vi "Main_maszyna.vi"() -> ()   [LabVIEW 2013]
doc: "Use this template to build a standard state machine design pattern. Each state executes code and determines which state to transition to. Contrast this design pattern with the User Interface Event Handler pattern, in which code executes in response to user actions. Contrast this design pattern also with the Queued Message Handler pattern, in which each message handling code can queue zero or more new messages.\nNote: This template does not contain the most recent programming guidelines recommended by National Instruments. For a complete, project-based implementation of the Standard State Machine pattern, use the Create Project dialog box instead of this template."
uses:
  inne pliki/Stany.ctl
  inne pliki/Params.ctl
  inne pliki/Data.ctl
panel:
  out "Warning text":string
  out "Warning":bool
  in  "Temp limits":T1={"Max (25)"=22.0, "Min (0)"=0.0}
  out "Waveform Chart":cluster{"Temperatura":dbl, "Średnia":dbl}(graph)
  in  "Akcje":T2
  out "Stan aktualny":T3
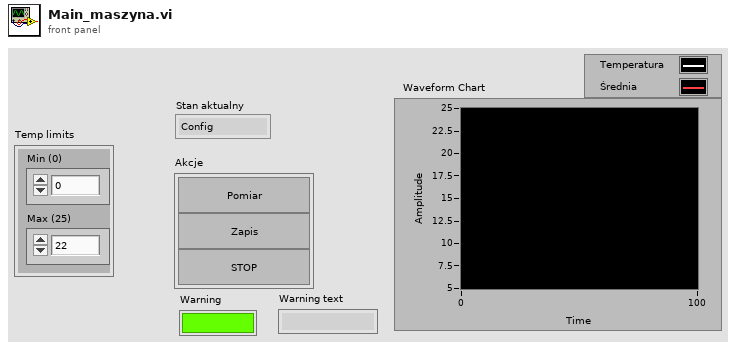
[diagram p1: front panel]
types:
  T1 = typedef "Params.ctl" = cluster{"Max (25)":dbl, "Min (0)":dbl}
  T2 = cluster{"bPomiar":bool, "bZapis":bool, "bSTOP":bool}
  T3 = typedef "Stany.ctl" = enum16{"Config", "IDLE", "Measure", "Analyze", "Display", "STOP", "Save"}
  T4 = typedef "Data.ctl" = cluster{"Temperatura":dbl, "Średnia":dbl, "Warning":bool, "Warning text ":string, "Temp limits":T1}
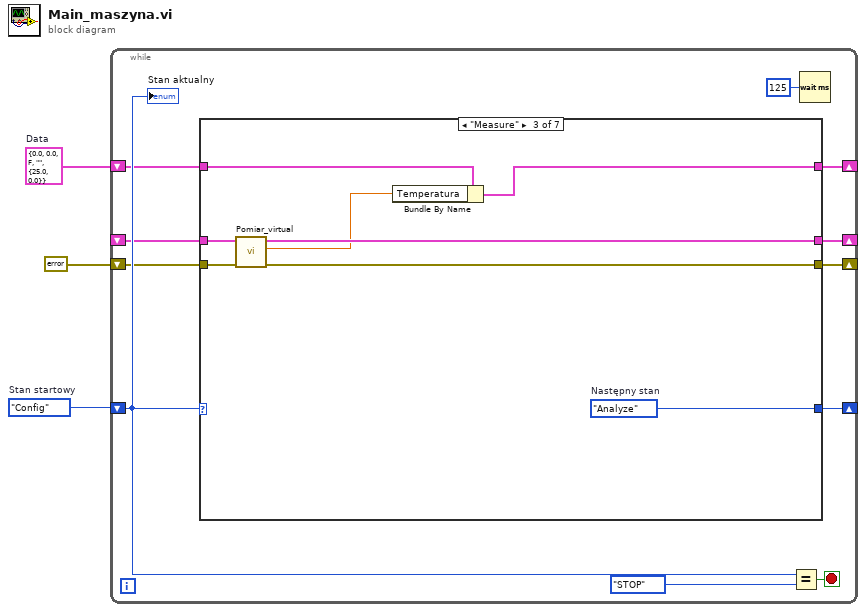
[diagram p0: block diagram]
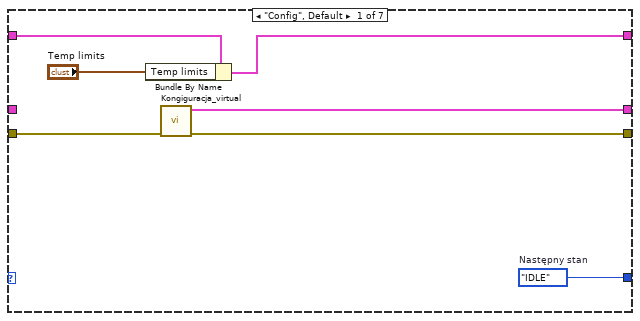
[diagram p2: hidden frame]
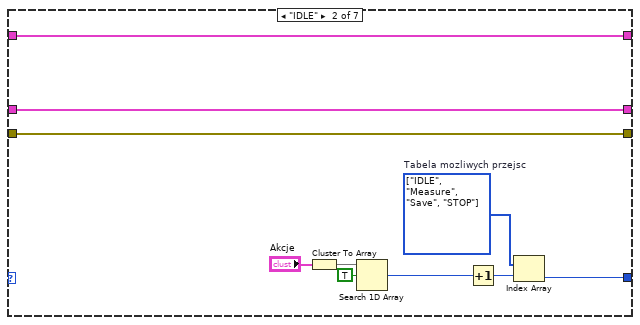
[diagram p3: hidden frame]
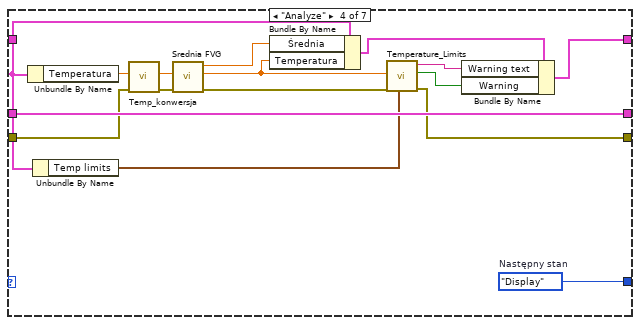
[diagram p4: hidden frame]
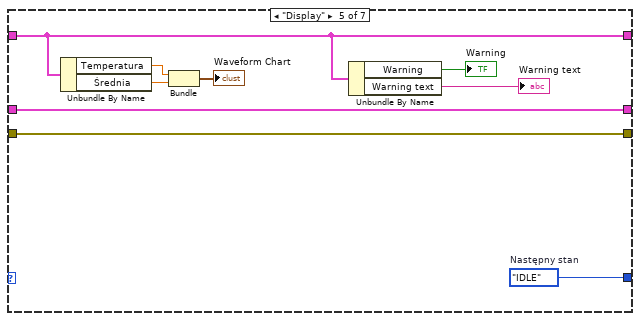
[diagram p5: hidden frame]
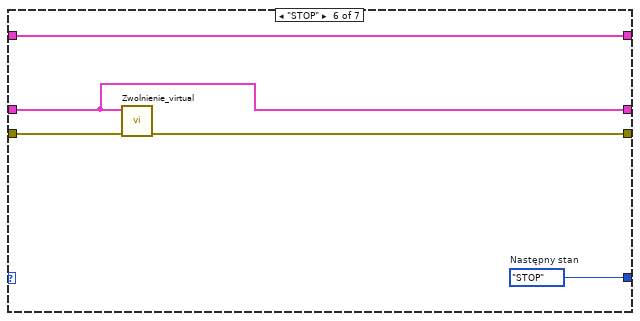
[diagram p6: hidden frame]
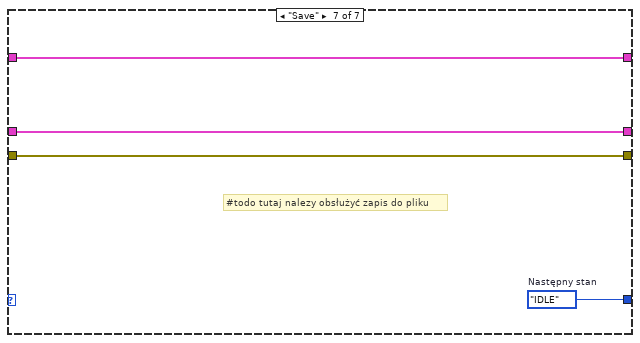
[diagram p7: hidden frame]
diagram:
  w2 = T4 {"Temperatura"=0.0, "Średnia"=0.0, "Warning"=FALSE, "Warning text "="", "Temp limits"={"Max (25)"=25.0, "Min (0)"=0.0}}  # Data
  w3 = Stany."Config"  # Stan startowy
  n1 = while {
    shift-right: [w12] -> _
    shift-left: w3 -> [w13]
    shift-right: [w8] -> _
    shift-left: w2 -> [w9]
    shift-right: [w7] -> _
    shift-left: _ -> [w6]
    shift-right: [w5] -> _
    shift-left: errorcluster {"status"=FALSE, "code"=0, "source"=""} ("error out") -> [w4]
    stop <- w14 stop-if-true
    n2 = case shown="\"Measure\"" w13 {
      tunnel: [w21 w26 w39 w55 w64 w69 w72] -> w12
      tunnel: w9 -> [w16 w24 w33 w51 w58 w68 w73]
      tunnel: [w15 w24 w32 w47 w58 w68 w73] -> w8
      tunnel: [w20 w23 w37 w54 w63 w65 w71] -> w7
      tunnel: w6 -> [_ w23 w38 w54 w63 w65 w71]
      tunnel: [w18 w22 w36 w45 w62 w66 w70] -> w5
      tunnel: w4 -> [w19 w22 w35 w46 w62 w67 w70]
      frame "Config", Default {
        w21 = Stany."IDLE"  # Następny stan
        n3 = Bundle By Name(cluster=w16, "Temp limits"="Temp limits") -> (w15:T4)
        n4 = call "Kongiguracja_virtual.vi"("error in (no error)"=w19) -> ("error out"=w18:errorcluster, "Reference out"=w20:cluster{"Numeric":dbl, "Boolean":bool})  [unwired: 9 in]
      }
      frame "IDLE" {
        w25 = T3[] [enum."IDLE", enum."Measure", enum."Save", enum."STOP"] items=["Config", "IDLE", "Measure", "Analyze", "Display", "STOP", "Save"]  # Tabela mozliwych przejsc
        n5 = Cluster To Array(cluster="Akcje") -> (array=w30:bool[])
        n6 = Search 1D Array(1D array=w30, element=TRUE) -> (index of element=w28:i32)  [unwired: 1 in]
        n7 = Increment(x=w28) -> (x+1=w27:i32)
        n8 = Index Array "Index Array"(array=w25, index=w27) -> (element=w26:T3)
      }
      frame "Measure" {
        w39 = Stany."Analyze"  # Następny stan
        n9 = call "Pomiar_virtual.vi"("error in (no error)"=w35, "Reference in"=w38) -> ("error out"=w36:errorcluster, "out"=w34:dbl, "Reference out"=w37:cluster{"Numeric":dbl, "Boolean":bool})  [unwired: 7 in]
        n10 = Bundle By Name(cluster=w33, "Temperatura"=w34) -> (w32:T4)
      }
      frame "Analyze" {
        w55 = Stany."Display"  # Następny stan
        n11 = Unbundle By Name(w51) -> ("Temperatura"=w53:dbl)
        n12 = Unbundle By Name(w51) -> ("Temp limits"=w52:T1)
        n13 = call "Temp_konwersja.vi"("error in (no error)"=w46, "Temp in"=w53) -> ("error out"=w44:errorcluster, "Temp out"=w43:dbl)  [unwired: 8 in]
        n14 = call "Srednia FVG.vi"("error in (no error)"=w44, "temperatura in"=w43) -> ("error out"=w42:errorcluster, "temperatura out"=w41:dbl, "średnia out"=w40:dbl)  [unwired: 7 in]
        n15 = Bundle By Name(cluster=w51, "Średnia"=w40, "Temperatura"=w41) -> (w48:T4)
        n16 = call "Temperature_Limits.vi"("Temp limits"=w52, "error in (no error)"=w42, "TEMP"=w41) -> ("error out"=w45:errorcluster, "Warning"=w49:bool, "Warning Text"=w50:string)  [unwired: 6 in]
        n17 = Bundle By Name(cluster=w48, "Warning text"=w50, "Warning"=w49) -> (w47:T4)
      }
      frame "Display" {
        w64 = Stany."IDLE"  # Następny stan
        n18 = Unbundle By Name(w58) -> ("Temperatura"=w60:dbl, "Średnia"=w61:dbl)
        n19 = Bundle("Temperatura"=w60, "Średnia"=w61) -> (→"Waveform Chart":cluster{"Temperatura":dbl, "Średnia":dbl})  [unwired: 1 in]
        n20 = Unbundle By Name(w58) -> ("Warning"=→"Warning":bool, "Warning text"=→"Warning text":string)
      }
      frame "STOP" {
        w69 = Stany."STOP"  # Następny stan
        n21 = call "Zwolnienie_virtual.vi"("error in (no error)"=w67, "Reference in"=w65) -> ("error out"=w66:errorcluster)  [unwired: 9 in]
      }
      frame "Save" {
        w72 = Stany."IDLE"  # Następny stan
        # "#todo tutaj nalezy obsłużyć zapis do pliku"
      }
    }
    n22 = Equal?(x=w13, y=Stany."STOP" ("Stan startowy")) -> (x = y?=w14:bool)
    n23 = Wait (ms)(milliseconds to wait=u32 125) -> ()  [unwired: 1 out]
    "Stan aktualny" <- w13
  }
